vi "FlpLib ResistorVtoI 2.vi"(1 "R":sgl, 5 "Vpos":sgl, 7 "Vneg":sgl) -> (6 "Current":sgl)   [LabVIEW 2017]
uses:
  <userlib>/_NI FLP Library/FPGA/outsideSCTL/FlpLib Subtract Shared Instance 2.vi
  <userlib>/_NI FLP Library/FPGA/outsideSCTL/FlpLib Divide Shared Instance 2.vi
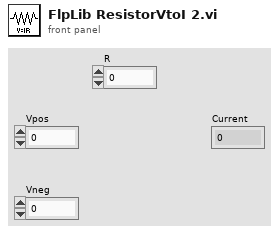
[diagram p1: front panel]
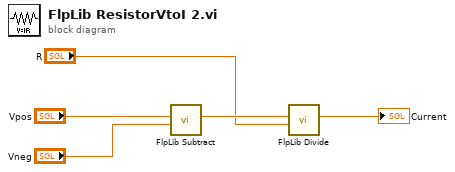
[diagram p0: block diagram]
diagram:
  n1 = call-poly <userlib>:"FlpLib Subtract.vi"("y"="Vneg", "x"="Vpos") -> ("x-y"=w3:sgl)  [unwired: 5 in]
  n2 = call-poly <userlib>:"FlpLib Divide.vi"("y"="R", "x"=w3) -> ("x/y"=→"Current":sgl)  [unwired: 5 in]
